vi "Prompt_message_no limit time.vi"(3 "error in":errorcluster, 5 "Message":string="Insert Unit and plug all cables, then press OK.") -> (0 "error out":errorcluster, 1 "Result":bool, 2 "Cancel":bool)   [LabVIEW 2015]
panel:
  out "UUT Sensor":bool
  in  "Cancel Task":string
  in  "Cancel Button":bool
  in  "Use Sensor":bool
  in  "Ok Task":string
  out "Timeout":bool
  out "Timer":u32
  in  "Timeout":i32=200000
  in  "OK Button":bool
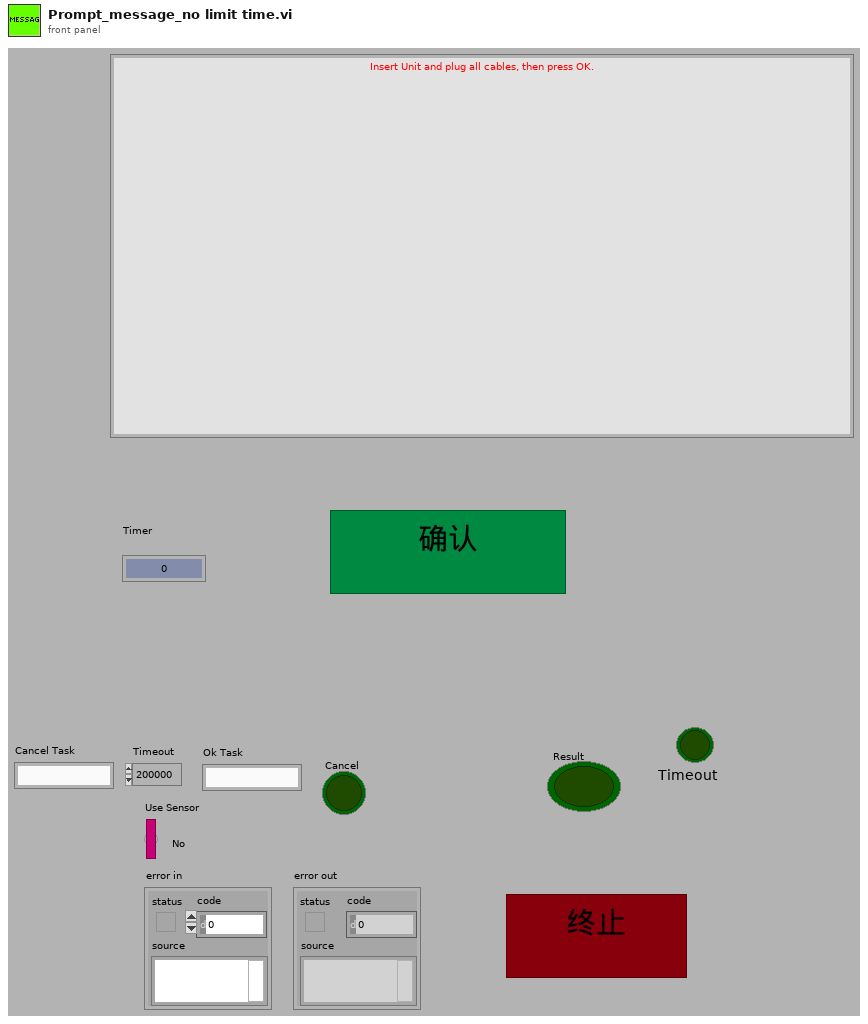
[diagram p1: front panel]
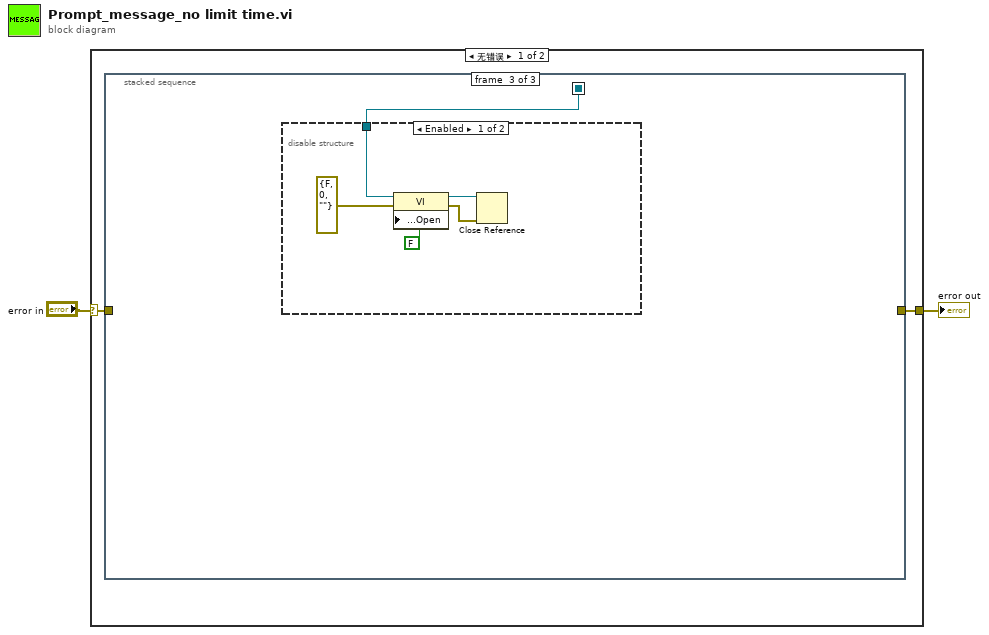
[diagram p0: block diagram]
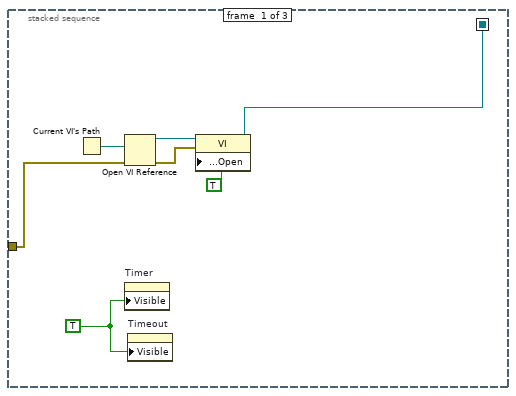
[diagram p2: hidden frame]
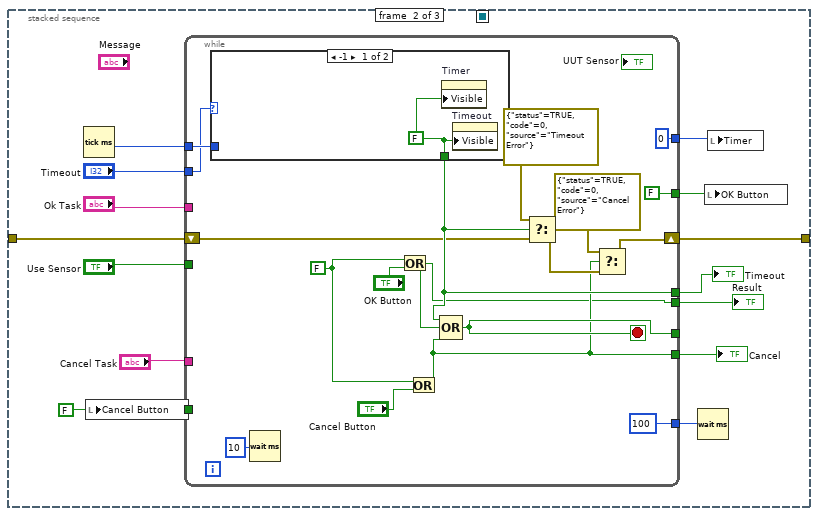
[diagram p3: hidden frame]
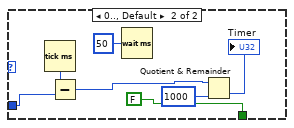
[diagram p4: hidden frame]
diagram:
  n1 = case shown="无错误" "error in" {
    selector: "error in" -> [w3 w58]
    tunnel: [w4 w58] -> w2
    frame No Error {
      n2 = stacked-sequence {
        seq-local: [w8 _ _] -> [_ _ w52]
        tunnel: [_ w25 _] -> w4
        tunnel: w3 -> [w5 w12 _]
        frame #0 {
          w6 = TRUE
          n3 = Current VI's Path() -> (path=w11:path)
          n4 = Open VI Reference(vi path=w11, error in (no error)=w5) -> (vi reference=w10:refnum<vi>, error out=w9:errorcluster)  [unwired: 4 in]
          n5 = property on="Timer" class="DigNum (严格)"("Visible"=w6) -> ()  [unwired: 2 in, 2 out]
          n6 = property on="Timeout" class="Bool (严格)"("Visible"=w6) -> ()  [unwired: 2 in, 2 out]
          n7 = property class="VI"(reference=w10, error in=w9, "Front Panel.Open"=TRUE ("Front Panel Window:Open")) -> (reference out=w8:refnum<vi>)  [unwired: 1 out]
        }
        frame #1 {
          w16 = FALSE
          n8 = Tick Count (ms)() -> (millisecond timer value=w23:u32)
          n9 = local write "Cancel Button"(w16) -> ()
          n10 = while {
            shift-right: [w34] -> w25
            shift-left: w12 -> [w28]
            tunnel: w23 -> [w43]
            tunnel: "Timeout" -> [w40]
            tunnel: [u32 0 ("y")] -> w22
            tunnel: [w37] -> w21
            tunnel: "Use Sensor" -> [_]
            tunnel: "Ok Task" -> [_]
            tunnel: [FALSE] -> w19
            tunnel: [w29] -> w17
            tunnel: w16 -> [_]
            tunnel: [w39] -> _
            tunnel: "Cancel Task" -> [_]
            tunnel: [u32 100 ("milliseconds to wait")] -> w14
            tunnel: [w27] -> w13
            stop <- w39 stop-if-true
            w26 = FALSE
            n11 = case shown="-1" w40 {
              tunnel: w43 -> [_ w50]
              tunnel: [w44 FALSE ("x > y?")] -> w37
              frame -1 {
                w44 = FALSE
                n12 = property on="Timer" class="DigNum (严格)"("Visible"=w44) -> ()  [unwired: 2 in, 2 out]
                n13 = property on="Timeout" class="Bool (严格)"("Visible"=w44) -> ()  [unwired: 2 in, 2 out]
              }
              frame 0.., Default {
                n14 = Tick Count (ms)() -> (millisecond timer value=w51:u32)
                n15 = Subtract(x=w51, y=w50) -> (x-y=w46:u32)
                n16 = Wait (ms)(milliseconds to wait=u32 50) -> ()  [unwired: 1 out]
                n17 = Quotient & Remainder(x=w46, y=u32 1000) -> (floor(x/y)=→"Timer":u32)  [unwired: 1 out]
              }
            }
            n18 = Wait (ms)(milliseconds to wait=u32 10) -> ()  [unwired: 1 out]
            n19 = Or(x=w26, y="OK Button") -> (x .or. y?=w27:bool)
            n20 = Or(x=w26, y="Cancel Button") -> (x .or. y?=w29:bool)
            n21 = Compound Arithmetic op=OR(w37, w27, w29) -> (w39:bool)
            n22 = Select(t=errorcluster {"status"=TRUE, "code"=0, "source"="Timeout Error"}, s=w37, f=w28) -> (s? t:f=w35:errorcluster)
            n23 = Select(t=errorcluster {"status"=TRUE, "code"=0, "source"="Cancel Error"}, s=w29, f=w35) -> (s? t:f=w34:errorcluster)
          }
          "Timeout" <- w21
          "Cancel" <- w17
          "Result" <- w13
          n24 = Wait (ms)(milliseconds to wait=w14) -> ()  [unwired: 1 out]
          n25 = local write "OK Button"(w19) -> ()
          n26 = local write "Timer"(w22) -> ()
        }
        frame #2 {
          n27 = disable-structure shown="Enabled" {
            disable-tunnel: w52 -> [w56 _]
            frame Enabled {
              n28 = property class="VI"(reference=w56, error in=errorcluster {"status"=FALSE, "code"=0, "source"=""} ("error in (no error)"), "Front Panel.Open"=FALSE ("Front Panel Window:Open")) -> (reference out=w55:refnum<vi>, error out=w54:errorcluster)
              n29 = Close Reference(reference=w55, error in (no error)=w54) -> ()  [unwired: 1 out]
            }
            frame Disabled {
            }
          }
        }
      }
    }
    frame Error {
    }
  }
  "error out" <- w2
